vi "Send PLC-Connection Status.vi"(7 "Message Priority (Normal)":T1=enum."Normal", 8 "error in (no error)":errorcluster, 9 "Remarks":string, 10 "Status":bool, 11 "Message Enqueuer":refnum<class "Message Enqueuer.lvclass">) -> (0 "error out":errorcluster, 3 "Message Enqueuer out":refnum<class "Message Enqueuer.lvclass">)   [LabVIEW 2022 SP3, in "PLCHandler - Controller -- Intefrace.lvlib" / "PLC-Connection Status Msg.lvclass"]
doc: "This VI sends the message to an actor."
uses:
  PLC-Connection Status Msg.lvclass
  PLC-Connection Status Msg.lvclass/PLC-Connection Status Msg.ctl
  <vilib>/ActorFramework/Message Enqueuer/Message Enqueuer.lvclass
  C:/Program Files/National Instruments/LabVIEW 2022/vi.lib/ActorFramework/Message/Message.lvclass
  E:/SourceCodes/image-harvest/PLCHandler - Controller -- Interface/PLCHandler - Controller -- Interface Messages/PLC-Connection Status Msg/PLC-Connection Status Msg.lvclass
  <vilib>/ActorFramework/Message Enqueuer/Message Priority.ctl
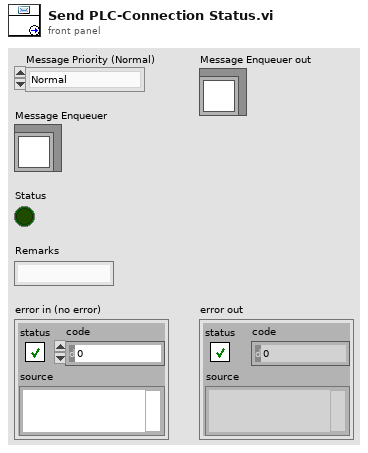
[diagram p1: front panel]
types:
  T1 = typedef "Actor Framework.lvlib/Message Enqueuer.lvclass/Message Priority.ctl" = enum16{"Low", "Normal", "High"}
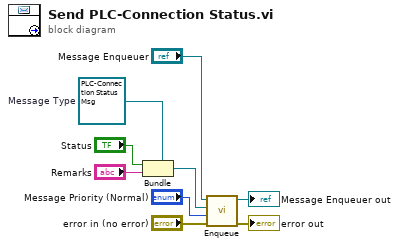
[diagram p0: block diagram]
diagram:
  w6 = refnum<class "PLC-Connection Status Msg.lvclass"> refnum  # Message Type
  n1 = Bundle(cluster=w6, "Status", "Remarks") -> (w5:refnum<class "PLC-Connection Status Msg.lvclass">)
  n2 = call <vilib>:"Enqueue.vi"("error in (no error)"="error in (no error)", "Message Priority (Normal)"="Message Priority (Normal)", "Message"=w5, "Message Enqueuer in"="Message Enqueuer") -> ("error out"=→"error out":errorcluster, "Message Enqueuer in"=→"Message Enqueuer out":refnum<class "Message Enqueuer.lvclass">)  [unwired: 6 in]
